vi "H5Lget_val (External).vi"(6 "lapl_id":T2, 8 "error in (no error)":errorcluster, 10 "Name":string=".", 11 "Location Ref":T2) -> (0 "error out":errorcluster, 1 "Object Path":string, 2 "Filename":path, 3 "Location Ref out":T2, 4 "type":T1 items=["H5L_TYPE_ERROR"=-1, "H5L_TYPE_HARD"=0, "H5L_TYPE_SOFT"=1, "H5L_TYPE_EXTERNAL"=64, "H5L_TYPE_MAX"=255])   [LabVIEW 2017]
doc: "Returns the value of a symbolic link."
uses:
  <vilib>/UPVI/lvhdf5/library.llb/HDF5 Ref.ctl
  <vilib>/UPVI/lvhdf5/link.llb/H5L_type_t.ctl
  <vilib>/UPVI/lvhdf5/error.llb/LVH5EMajorID.ctl
  <vilib>/UPVI/lvhdf5/error.llb/LVH5EMinorID.ctl
  <vilib>/UPVI/lvhdf5/error.llb/H5Epush_enum_enum.vi
panel:
  # "LVHDF5 Toolkit\nCopyright (c) 2005-2013 by Jason D. Sommerville\nCopyright (c) 2014-2015 by UPVI, LLC.\n\nThis use and distribution of this file is governed by the terms found in \nLICENSE.txt distributed with this toolkit and installed at\n <user.lib>\\_lvhdf5\\LICENSE.txt"
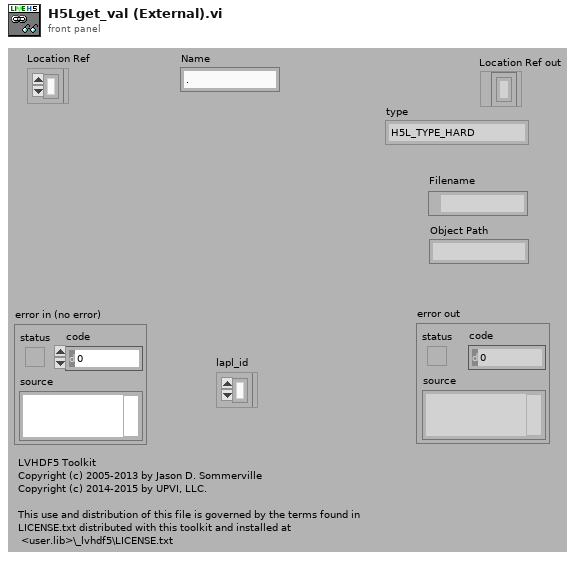
[diagram p1: front panel]
types:
  T1 = typedef "H5L_type_t.ctl" = i32
  T2 = typedef "HDF5 Ref.ctl" = refnum<k1>
  T3 = typedef "LVH5EMinorID.ctl" = string
  T4 = typedef "LVH5EMajorID.ctl" = string
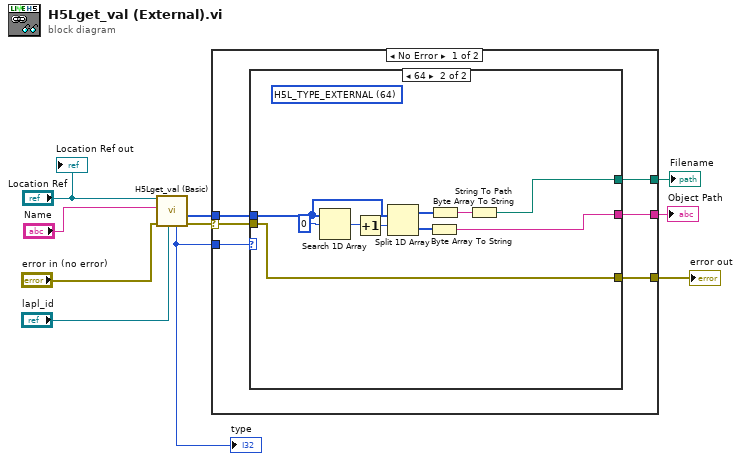
[diagram p0: block diagram]
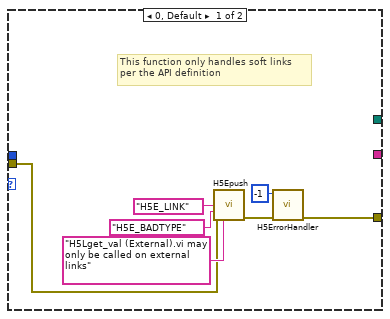
[diagram p2: hidden frame]
diagram:
  n1 = call <vilib>:"H5Lget_val (Basic).vi"("lapl_id"="lapl_id", "error in (no error)"="error in (no error)", "Name"="Name", "Location Ref"="Location Ref") -> ("error out"=w7:errorcluster, "buffer"=w6:u8[], "type"=w2:T1)  [unwired: 4 in, 1 out]
  "type" <- w2
  n2 = case shown="No Error" w7 {
    selector: w7 -> [w14 w34]
    tunnel: w6 -> [w16 _]
    tunnel: [w15 _] -> w4
    tunnel: [w13 w34] -> w5
    tunnel: [w12 _] -> w3
    tunnel: w2 -> [w11 _]
    frame No Error {
      n3 = case shown="64" w11 {
        tunnel: w16 -> [_ w29]
        tunnel: [_ w24] -> w15
        tunnel: w14 -> [w18 w33]
        tunnel: [w17 w33] -> w13
        tunnel: [_ w25] -> w12
        frame 0, Default {
          # "This function only handles soft links\nper the API definition"
          n4 = call-poly <vilib>:"H5Epush.vi"("major_id"=T4 "H5E_LINK", "minor_id"=T3 "H5E_BADTYPE", "error in (no error)"=w18, "msg"="H5Lget_val (External).vi may only be called on external links") -> ("error out"=w20:errorcluster)  [unwired: 10 in, 1 out]
          n5 = call <vilib>:"H5ErrorHandler.vi"("error in (no error)"=w20, "herr_t"=-1) -> ("error out"=w17:errorcluster)  [unwired: 3 in, 4 out]
        }
        frame 64 {
          (unwired) T1 64 items=["H5L_TYPE_ERROR"=-1, "H5L_TYPE_HARD"=0, "H5L_TYPE_SOFT"=1, "H5L_TYPE_EXTERNAL"=64, "H5L_TYPE_MAX"=255] ("type")
          n6 = Search 1D Array(1D array=w29, element=u8 0) -> (index of element=w31:i32)  [unwired: 1 in]
          n7 = Increment(x=w31) -> (x+1=w30:i32)
          n8 = Split 1D Array(array=w29, index=w30) -> (first subarray=w27:u8[], second subarray=w28:u8[])
          n9 = Byte Array To String(unsigned byte array=w28) -> (string=w24:string)
          n10 = Byte Array To String(unsigned byte array=w27) -> (string=w26:string)
          n11 = String To Path(string=w26) -> (path=w25:path)
        }
      }
    }
    frame Error {
    }
  }
  "error out" <- w5
  "Object Path" <- w4
  "Filename" <- w3
  "Location Ref out" <- "Location Ref"
